vi "flashOpen.vi"   [LabVIEW 2017]
uses:
  globalDevices.vi
  <vilib>/DAQmx/create/channels.llb/DAQmx Create Channel (DO-Digital Output).vi
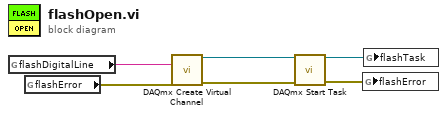
[diagram p0: block diagram]
diagram:
  n1 = global read "globalDevices.vi" "flashDigitalLine"() -> (w6:tag)
  n2 = global read "globalDevices.vi" "flashError"() -> (w5:errorcluster)
  n3 = call-poly <vilib>:"DAQmx Create Virtual Channel.vi"("lines"=w6, "error in"=w5) -> ("task out"=w4:refnum<k21>, "error out"=w3:errorcluster)  [unwired: 12 in]
  n4 = call <vilib>:"DAQmx Start Task.vi"("task/channels in"=w4, "error in"=w3) -> ("task out"=w2:refnum<k21>, "error out"=w1:errorcluster)  [unwired: 12 in]
  n5 = global write "globalDevices.vi" "flashError"(w1) -> ()
  n6 = global write "globalDevices.vi" "flashTask"(w2) -> ()
